vi "ALTS-2015 Init All.vi"(8 "error in":errorcluster) -> (0 "error out":errorcluster)   [LabVIEW 2013]
doc: "Copyright © 2005, Soliton Technologies.\nAll rights reserved."
uses:
  Controls/ALTS-2015 LV2GBL Station Info Options.ctl
  Controls/ALTS-2015 Write DB Write Result Driver Cases.ctl
  Controls/ALTS-2015 Obtain Test Data DB Driver Options.ctl
  Controls/ALTS-2015 LV2GBL Options.ctl
  Controls/ALTS-2015 Scanner Driver Options.ctl
  Controls/ALTS-2015 DB Driver Options.ctl
  Controls/ALTS-2015 LV2GBL WorkOrder&SN Info Options.ctl
  SLL DAQ Engine/Software/Source Code/Sub VIs/DAQ Engine/Controls/SLL DE DO Command LV2Global Options.ctl
  SLL DAQ Engine/Software/Source Code/Sub VIs/DAQ Engine/Controls/SLL DE DO Global Options.ctl
  SLL DAQ Engine/Software/Source Code/Sub VIs/DAQ Engine/Controls/SLL DE DI Global Options.ctl
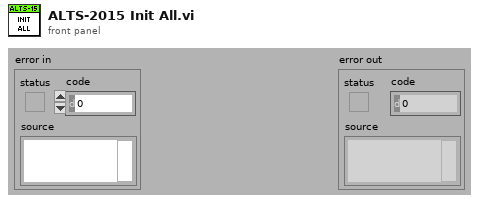
[diagram p1: front panel]
types:
  T1 = typedef "ALTS-2015 LV2GBL WorkOrder&SN Info Options.ctl" = enum16{"Init", "Read all", "Write Work Order"}
  T2 = typedef "ALTS-2015 DB Driver Options.ctl" = enum16{"Init", "Read DB", "Close"}
  T3 = typedef "ALTS-2015 LV2GBL Options.ctl" = enum16{"Read all", "Write all"}
  T4 = typedef "ALTS-2015 Scanner Driver Options.ctl" = enum16{"Initialize Scanner", "Read Scanner", "Close Scanner"}
  T5 = typedef "ALTS-2015 Obtain Test Data DB Driver Options.ctl" = enum16{"Init", "Read Test Data Results", "Close"}
  T6 = typedef "ALTS-2015 Write DB Write Result Driver Cases.ctl" = enum16{"Init", "Write Result", "Close"}
  T7 = typedef "ALTS-2015 LV2GBL Station Info Options.ctl" = enum16{"Init", "Read", "Read All", "Write Sensor ID", "Write  Work Order", "Write Serial Number", "Write Test Data", "Write Station Status", "Write Station Occupancy", "Write Station Test Type", "Write Rerun", "Write Load Decision", "Clear All", "Clear Test Result"}
  T8 = typedef "SLL DE DI Global Options.ctl" = enum16{"Init", "Write Line", "Write Array", "Read Line", "Read Array", "Read Full Status", "Write Full Status"}
  T9 = typedef "SLL DE DO Global Options.ctl" = enum16{"Init", "Write Line", "Write Array", "Write Full Status", "Read Line", "Read Array", "Read Full Status", "Restart DO", "Send to Safe Mode", "Stop DO"}
  T10 = typedef "SLL DE DO Command LV2Global Options.ctl" = enum16{"Init/Register Events", "Get Event Refnum", "Fire Event", "Destroy Event"}
  T11 = typedef "ALTS-2015 INI Configuration Cluster.ctl" = cluster{"Application":cluster{"Rerun Count":i32, "Workorder No":string}, "Station Details":cluster{"Sensor Name 1":string, "Sensor Name 2":string, "Sensor Name 3":string, "Sensor Name 4":string, "Station1 Enable":bool, "Station2 Enable":bool, "Station3 Enable":bool, "Station4 Enable":bool}, "Database":cluster{"Database Connection Link":path, "Result Procedure":string, "User":string, "Password":string, "Prompt":bool, "Station 1 LT Result DB DSN Path":path, "Station 2 LT Result DB DSN Path":path, "Station 3 LT Result DB DSN Path":path, "Station 4 LT Result DB DSN Path":path, "AirLeakTestResult Procedure":string, "Serial Details Procedure":string}, "Simulation":cluster{"Simulate DAQ Hardware":bool, "Simulate Result DB Write":bool, "Simulate Scanner":bool, "Simulate OPC":bool, "Simulate Serial Details DB":bool, "Simulate Result DB":bool, "Simulate Scanner DB Path":path, "Simulate Serial Details DB Path":path, "Simulate Result DB Path":path}, "Barcode Scanner1":cluster{"Scanner IP":string, "Scanner Port":u16, "#Bytes to Read":i32}, "Barcode Scanner2":cluster{"Enabled?":bool, "Scanner IP":string, "Scanner Port":u16, "#Bytes to Read":i32}}
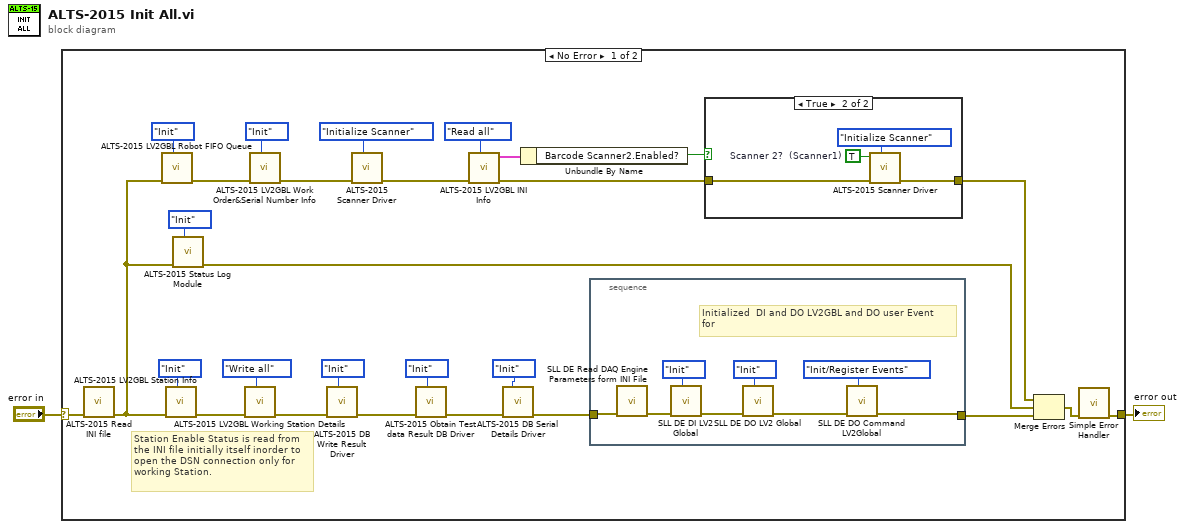
[diagram p0: block diagram]
diagram:
  n1 = case shown="No Error" "error in" {
    selector: "error in" -> [w30 w44]
    tunnel: [w22 w44] -> w1
    frame No Error {
      # "Station Enable Status is read from the INI file initially itself inorder to open the DSN connection only for working Station."
      n2 = call "ALTS-2015 Read INI file.vi"("error in (no error)"=w30) -> ("error out"=w4:errorcluster)  [unwired: 10 in]
      n3 = call "ALTS-2015 LV2GBL Robot FIFO Queue.vi"("Enum"=enum16{"Init", "Enqueue", "Dequeue", "Destroy"}."Init", "error in (no error)"=w4) -> ("error out"=w7:errorcluster)  [unwired: 7 in, 2 out]
      n4 = call "ALTS-2015 LV2GBL Station Info.vi"("Options"=ALTS-2015_LV2GBL_Station_Info_Options."Init", "error in"=w4) -> ("error out"=w24:errorcluster)  [unwired: 5 in, 4 out]
      n5 = call "ALTS-2015 Status Log Module.vi"("Options"=enum16{"Init", "Write", "Close"}."Init", "error in"=w4) -> ("error out"=w3:errorcluster)  [unwired: 9 in]
      n6 = call "ALTS-2015 LV2GBL Working Station Details.vi"("Options"=ALTS-2015_LV2GBL_Options."Write all", "error in"=w24) -> ("error out"=w23:errorcluster)  [unwired: 8 in, 1 out]
      n7 = call "ALTS-2015 LV2GBL Work Order&Serial Number Info.vi"("Options"=ALTS-2015_LV2GBL_WorkOrder&SN_Info_Options."Init", "error in"=w7) -> ("error out"=w6:errorcluster)  [unwired: 8 in, 1 out]
      n8 = call "ALTS-2015 DB Write Result Driver.vi"("Operation"=ALTS-2015_Write_DB_Write_Result_Driver_Cases."Init", "Error In"=w23) -> ("error out"=w29:errorcluster)  [unwired: 9 in]
      n9 = call "ALTS-2015 Scanner Driver.vi"("Operation"=ALTS-2015_Scanner_Driver_Options."Initialize Scanner", "error in (no error)"=w6) -> ("error out"=w19:errorcluster)  [unwired: 8 in, 1 out]
      n10 = call "ALTS-2015 Obtain Test data Result DB Driver.vi"("Option"=ALTS-2015_Obtain_Test_Data_DB_Driver_Options."Init", "error in"=w29) -> ("error out"=w12:errorcluster)  [unwired: 8 in, 1 out]
      n11 = call "ALTS-2015 LV2GBL INI Info.vi"("Options"=ALTS-2015_LV2GBL_Options."Read all", "error in"=w19) -> ("error out"=w17:errorcluster, "Configuration Cluster Out"=w18:T11)  [unwired: 8 in]
      n12 = call "ALTS-2015 DB Serial Details Driver.vi"("Operation"=ALTS-2015_DB_Driver_Options."Init", "error in (no error)"=w12) -> ("error out"=w9:errorcluster)  [unwired: 11 in, 2 out]
      n13 = Unbundle By Name(w18) -> ("Barcode Scanner2.Enabled?"=w16:bool)
      n14 = stacked-sequence {
        tunnel: w9 -> [w37]
        tunnel: [w36] -> w25
        frame #0 {
          # "Initialized  DI and DO LV2GBL and DO user Event\nfor"
          n15 = call "SLL DE Read DAQ Engine Parameters form INI File.vi"("error in (no error)"=w37) -> ("error out"=w41:errorcluster)  [unwired: 10 in]
          n16 = call "SLL DE DI LV2 Global.vi"("Option"=SLL_DE_DI_Global_Options."Init", "error in (no error)"=w41) -> ("error out"=w42:errorcluster)  [unwired: 6 in, 3 out]
          n17 = call "SLL DE DO LV2 Global.vi"("DO Option"=SLL_DE_DO_Global_Options."Init", "Error In"=w42) -> ("error out"=w43:errorcluster)  [unwired: 6 in, 3 out]
          n18 = call "SLL DE DO Command LV2Global.vi"("Option"=SLL_DE_DO_Command_LV2Global_Options."Init/Register Events", "Error in (no error)"=w43) -> ("Error out"=w36:errorcluster)  [unwired: 8 in, 1 out]
        }
      }
      n19 = case shown="True" w16 {
        tunnel: w17 -> [w31 w34]
        tunnel: [w31 w32] -> w14
        frame False {
        }
        frame True {
          w33 = TRUE  # Scanner 2?  (Scanner1)
          n20 = call "ALTS-2015 Scanner Driver.vi"("Operation"=ALTS-2015_Scanner_Driver_Options."Initialize Scanner", "error in (no error)"=w34, "Scanner 2?  (Scanner1)"=w33) -> ("error out"=w32:errorcluster)  [unwired: 7 in, 1 out]
        }
      }
      n21 = Merge Errors(w14, w3, w25) -> (w15:errorcluster)
      n22 = call <vilib>:"Simple Error Handler.vi"("error in (no error)"=w15) -> ("error out"=w22:errorcluster)  [unwired: 4 in, 4 out]
    }
    frame Error {
    }
  }
  "error out" <- w1
